vi "Internal Close.vi"(1 "Interface TypeDefs":T1 {"I2CDevRef"."Device Address" format="%.0x"}, 2 "navX Device":T8={"Interface"={"Protocol"=enum."SERIAL", "Update Rate (4Hz-60Hz)"=4, "navX Open TypeDef"=variant}, "Notifiy Packet"=refnum, "Loop VI Refnum"=refnum} {"Interface"."Update Rate (4Hz-60Hz)" min=4 max=60 step=1}) -> (0 "error out":errorcluster)   [LabVIEW 2014, in "navX Library v2.lvlib"]
uses:
  navX Library v2.lvlib
  TypeDefs/navX Device TypeDef.ctl
  TypeDefs/navX Protocol TypeDef.ctl
  TypeDefs/navX Notify Packet TypeDef.ctl
  TypeDefs/navX Action TypeDef.ctl
  TypeDefs/navX Interface TypeDef.ctl
  <vilib>/Rock Robotics/WPI/SerialPort/WPI_SerialPortRef.ctl
  <vilib>/Rock Robotics/WPI/I2C/WPI_I2CDevRef.ctl
  <vilib>/Rock Robotics/SystemInterfaces/Typedef/FPGA_TypedefDigitalModule.ctl
  <vilib>/Rock Robotics/SystemInterfaces/i2clib/i2c_bus.ctl
  <vilib>/Rock Robotics/WPI/SPI/WPI_SPIDevRef.ctl
  <vilib>/Rock Robotics/SystemInterfaces/spilib/spi_bus.ctl
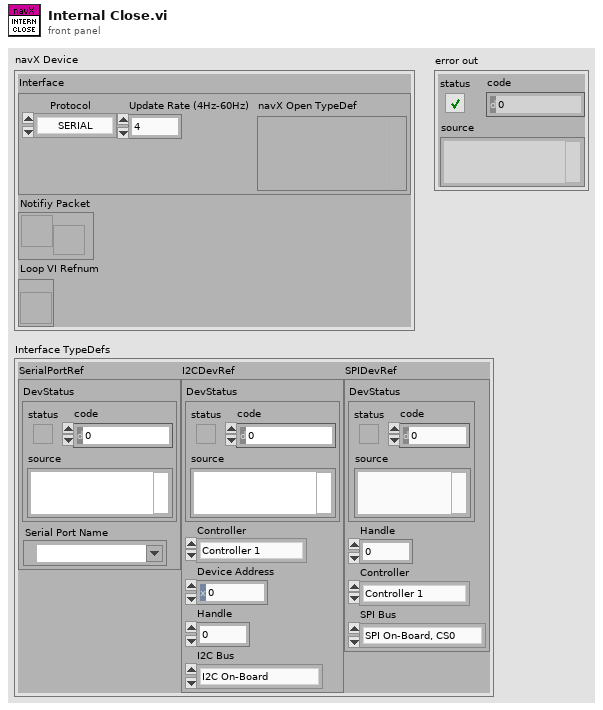
[diagram p1: front panel]
types:
  T1 = typedef "navX Library v2.lvlib/navX Interface TypeDef.ctl" = cluster{"SerialPortRef":T2, "I2CDevRef":T3, "SPIDevRef":T6}
  T2 = typedef "WPI_SerialPortRef.ctl" = cluster{"DevStatus":errorcluster, "Serial Port Name":refnum<visa-resource-name>}
  T3 = typedef "WPI_I2CDevRef.ctl" = cluster{"DevStatus":errorcluster, "Controller":T4, "Device Address":u8, "Handle":i32, "I2C Bus":T5}
  T4 = typedef "FPGA_TypedefDigitalModule.ctl" = enum16{"Controller 1"}
  T5 = typedef "i2c_bus.ctl" = enum16{"I2C On-Board", "I2C MXP", "Invalid"}
  T6 = typedef "WPI_SPIDevRef.ctl" = cluster{"DevStatus":errorcluster, "Handle":i32, "Controller":T4, "SPI Bus":T7}
  T7 = typedef "spi_bus.ctl" = enum16{"SPI On-Board, CS0", "SPI On-Board, CS1", "SPI On-Board, CS2", "SPI On-Board, CS3", "SPI MXP", "Invalid"}
  T8 = typedef "navX Library v2.lvlib/navX Device TypeDef.ctl" = cluster{"Interface":cluster{"Protocol":T9, "Update Rate (4Hz-60Hz)":u8, "navX Open TypeDef":variant}, "Notifiy Packet":refnum<notifier>, "Loop VI Refnum":refnum<vi>}
  T9 = typedef "navX Library v2.lvlib/navX Protocol TypeDef.ctl" = enum16{"SERIAL", "I2C", "SPI"}
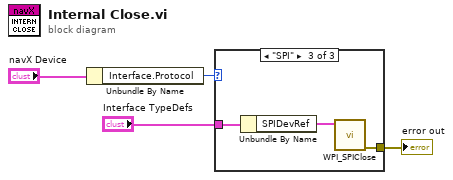
[diagram p0: block diagram]
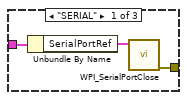
[diagram p2: hidden frame]
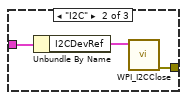
[diagram p3: hidden frame]
diagram:
  n1 = Unbundle By Name("navX Device") -> ("Interface.Protocol"=w1:T9)
  n2 = case shown="\"SPI\"" w1 {
    tunnel: "Interface TypeDefs" -> [w7 w10 w13]
    tunnel: [w5 w8 w11] -> w4
    frame "SERIAL" {
      n3 = Unbundle By Name(w7) -> ("SerialPortRef"=w6:T2)
      n4 = call <vilib>:"WPI_SerialPortClose.vi"("SerialPortRef"=w6) -> ("error out"=w5:errorcluster)  [unwired: 10 in]
    }
    frame "I2C" {
      n5 = Unbundle By Name(w10) -> ("I2CDevRef"=w9:T3)
      n6 = call <vilib>:"WPI_I2CClose.vi"("I2CDevRef"=w9) -> ("error out"=w8:errorcluster)  [unwired: 10 in]
    }
    frame "SPI" {
      n7 = Unbundle By Name(w13) -> ("SPIDevRef"=w12:T6)
      n8 = call <vilib>:"WPI_SPIClose.vi"("SPIDevRef"=w12) -> ("error out"=w11:errorcluster)  [unwired: 10 in]
    }
  }
  "error out" <- w4
